vi "FTW-Endpoint-Ask.vi"(0 "FTW Socket":refnum<class "FTW-Endpoint.lvclass">, 5 "Request Header":string, 7 "Request Body":string, 9 "Timeout":i32 format="%dmsec", 11 "error in":errorcluster) -> (4 "FTW Socket out":refnum<class "FTW-Endpoint.lvclass">, 6 "Response Header":string, 8 "Response Body":string, 10 "Timed out?":bool, 15 "error out":errorcluster)   [LabVIEW 2013, in "FTW-Actor.lvlib" / "FTW-Endpoint.lvclass"]
uses:
  FTW-Endpoint.lvclass
  Request/FTW-Request.lvclass
panel:
  # "Inputs"
  # "Outputs"
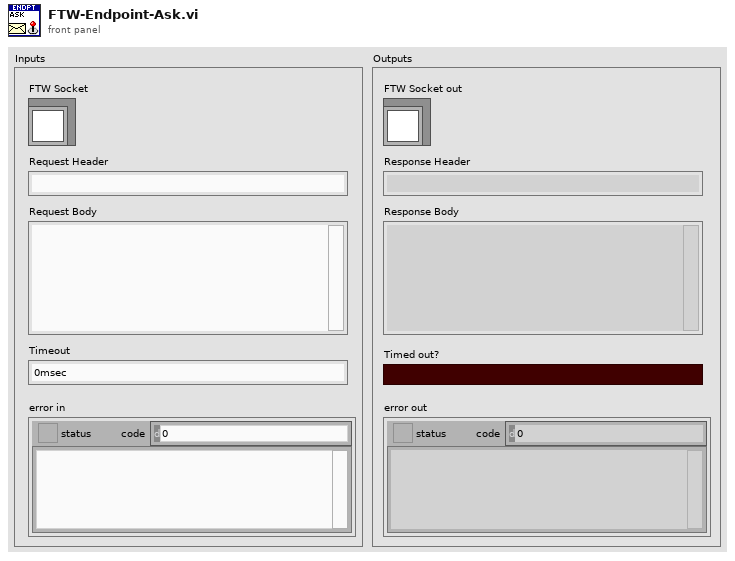
[diagram p1: front panel]
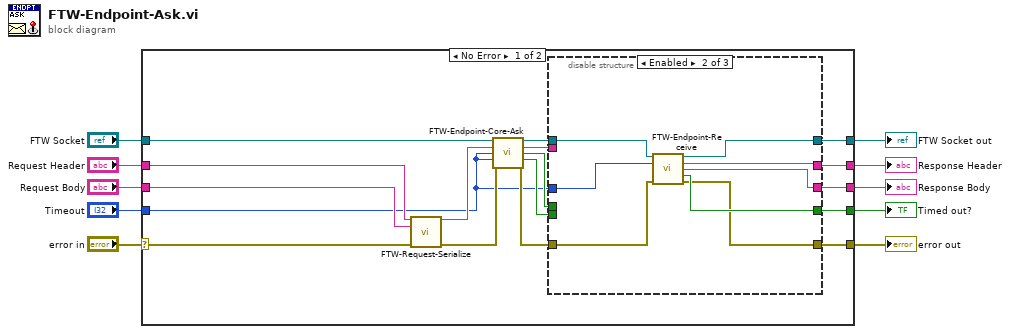
[diagram p0: block diagram]
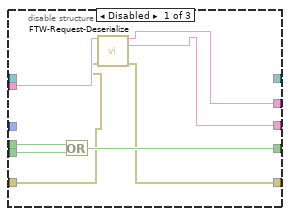
[diagram p2: hidden frame]
diagram:
  n1 = case shown="No Error" "error in" {
    selector: "error in" -> [w16 w47]
    tunnel: [w19 w47] -> w10
    tunnel: [w17 w46] -> w8
    tunnel: "FTW Socket" -> [w27 w46]
    tunnel: [w24 _] -> w6
    tunnel: "Timeout" -> [w11 _]
    tunnel: "Request Header" -> [w13 _]
    tunnel: "Request Body" -> [w12 _]
    tunnel: [w22 _] -> w2
    tunnel: [w21 _] -> w1
    frame No Error {
      n2 = call "FTW-Request-Serialize.vi"("Request Header"=w13, "Request Body"=w12, "error in"=w16) -> ("Request"=w15:string, "error out"=w14:errorcluster)  [unwired: 11 in]
      n3 = call "FTW-Endpoint-Core-Ask.vi"("FTW Socket"=w27, "Request"=w15, "Read Timeout"=w11, "Write Timeout"=w11, "error in"=w14) -> ("FTW Socket out"=w18:refnum<class "FTW-Endpoint.lvclass">, "Response"=w23:string, "Read Timed out?"=w26:bool, "Write Timed out?"=w25:bool, "error out"=w20:errorcluster)  [unwired: 6 in]
      n4 = disable-structure shown="Enabled" {
        disable-tunnel: w26 -> [w35 _ _]
        disable-tunnel: w25 -> [w34 _ _]
        disable-tunnel: [w33 w39 _] -> w24
        disable-tunnel: w23 -> [w32 _ _]
        disable-tunnel: [w29 w41 _] -> w22
        disable-tunnel: [w28 w40 _] -> w21
        disable-tunnel: w20 -> [w31 w37 w44]
        disable-tunnel: [w30 w36 w44] -> w19
        disable-tunnel: w18 -> [_ w43 w45]
        disable-tunnel: [_ w42 w45] -> w17
        disable-tunnel: w11 -> [_ w38 _]
        frame Disabled {
          n5 = Or(x=w35, y=w34) -> (x .or. y?=w33:bool)
          n6 = call "FTW-Request-Deserialize.vi"("Message"=w32, "error in"=w31) -> ("Message Header"=w29:string, "Message Body"=w28:string, "error out"=w30:errorcluster)  [unwired: 11 in]
        }
        frame Enabled {
          n7 = call-dynamic "FTW-Endpoint-Receive.vi"("FTW Endpoint"=w43, "Timeout"=w38, "error in"=w37) -> ("FTW Endpoint out"=w42:refnum<class "FTW-Endpoint.lvclass">, "Message Header"=w41:string, "Response Body"=w40:string, "Timed out?"=w39:bool, "error out"=w36:errorcluster)  [unwired: 8 in]
        }
        frame Disabled {
        }
      }
    }
    frame Error {
    }
  }
  "error out" <- w10
  "FTW Socket out" <- w8
  "Timed out?" <- w6
  "Response Header" <- w2
  "Response Body" <- w1
